vi "Initialize Modbus Slave Connection.vi"(8 "error in (no error)":errorcluster, 11 "Parameters":T1={"Interface Data"={"Name"="", "Unit ID"=0, "Refresh Rate"=0, "Write Rate"=0, "Write Mode"=enum."Value Change", "Interface Type"=enum."TCP Master", "TCP Settings"={"Address"="", "Port"=0, "Timeout"=0}, "Serial Settings"={"VISA resource name"="", "baud rate"=0, "parity (even)"=0, "flow control (none)"=0, "serial type"=enum."RTU", "Wire Mode"=-1}}, "Modbus Input Groups"=[], "Modbus Output Groups"=[], "error in (no error)"={"status"=FALSE, "code"=0, "source"=""}, "Modbus Input Engine Group Names"=[], "Modbus Output Engine Group Names"=[]} {"Interface Data"."Serial Settings"."Wire Mode" items=["Unknown"=-1, "RS485/Wire4"=0, "RS485/Wire2-EchoDTR"=1, "RS485/Wire2-CtrlDTR"=2, "RS485/Wire2-Auto"=3, "RS232/DTE"=128, "RS232/DCE"=129, "RS232/AUTO"=130]; "Interface Data"."Serial Settings"."parity (even)" items=["None", "Odd", "Even", "Mark", "Space"]; "Interface Data"."Serial Settings"."flow control (none)" items=["None", "XON/XOFF", "RTS/CTS", "XON/XOFF & RTS/CTS", "DTR/DSR", "XON/XOFF & DTR/DSR"]}) -> (0 "error out":errorcluster, 3 "Modbus Slave Out":refnum<class "Modbus Slave.lvclass">)   [LabVIEW 2021, in "Modbus Master Engine.lvlib"]
uses:
  Modbus Master Engine.lvlib
  Shared/Device Info.ctl
  Shared/Write Mode.ctl
  Shared/Controls/Interface Type.ctl
  Shared/Controls/Data Model/TCP Settings.ctl
  Shared/Controls/Data Model/Serial Settings.ctl
  Bulk Data Access.ctl
  System Explorer/SubVIs/Modbus Type.ctl
  Shared/Controls/Data Model/Channel.ctl
  <vilib>/NI VeriStand/Custom Device API/Custom Device Channel Type.ctl
  Shared/Controls/Data Model/Mapping.ctl
  Shared/Controls/Data Model/DataType.ctl
  <vilib>/NI VeriStand/Custom Device API/Custom Device Item Ref.ctl
  Modbus API.lvlibp/API/Slave/Modbus Slave.lvclass
  Modbus API.lvlibp/API/Wrapper/API Main.lvlib
  Shared/Modbus Master Shared.lvlib
  <vilib>/NI VeriStand/Custom Device API/Custom Device API.lvlib
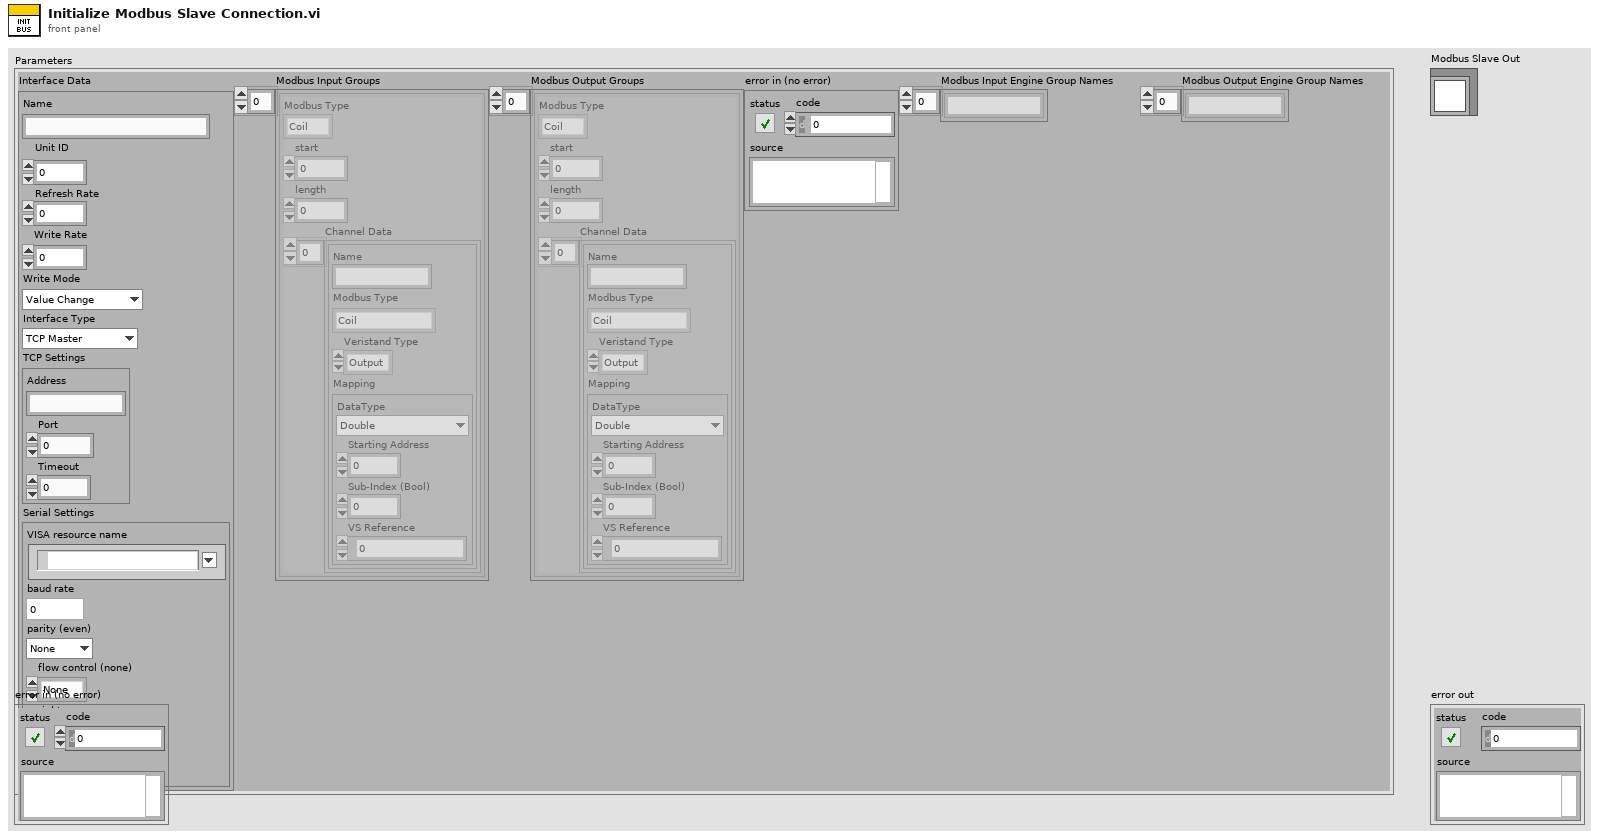
[diagram p1: front panel]
types:
  T1 = typedef "Modbus Master Shared.lvlib/Device Info.ctl" = cluster{"Interface Data":cluster{"Name":string, "Unit ID":u8, "Refresh Rate":i32, "Write Rate":i32, "Write Mode":T2, "Interface Type":T3, "TCP Settings":T4, "Serial Settings":T5}, "Modbus Input Groups":T6[], "Modbus Output Groups":T6[], "error in (no error)":errorcluster, "Modbus Input Engine Group Names":string[], "Modbus Output Engine Group Names":string[]}
  T2 = typedef "Modbus Master Shared.lvlib/Write Mode.ctl" = enum16{"Value Change", "Interval"}
  T3 = typedef "Modbus Master Shared.lvlib/Interface Type.ctl" = enum16{"TCP Master", "Serial Master", "TCP Slave", "Serial Slave"}
  T4 = typedef "Modbus Master Shared.lvlib/TCP Settings.ctl" = cluster{"Address":string, "Port":u16, "Timeout":i32}
  T5 = typedef "Modbus Master Shared.lvlib/Serial Settings.ctl" = cluster{"VISA resource name":refnum<visa-resource-name>, "baud rate":u32, "parity (even)":u16, "flow control (none)":u16, "serial type":enum16{"RTU", "ASCII"}, "Wire Mode":i16}
  T6 = typedef "Modbus Master Shared.lvlib/Bulk Data Access.ctl" = cluster{"Modbus Type":T7, "start":u16, "length":u16, "Channel Data":T8[]}
  T7 = typedef "Modbus Master Shared.lvlib/Modbus Type.ctl" = enum16{"Coil", "Discrete Input", "Holding Register", "Input Register"}
  T8 = typedef "Modbus Master Shared.lvlib/Channel.ctl" = cluster{"Name":string, "Modbus Type":T7, "Veristand Type":T9, "Mapping":T10}
  T9 = typedef "Custom Device API.lvlib/Custom Device Channel Type.ctl" = enum16{"Input", "Output"}
  T10 = typedef "Modbus Master Shared.lvlib/Mapping.ctl" = cluster{"DataType":T11, "Starting Address":u16, "Sub-Index (Bool)":u16, "VS Reference":T12}
  T11 = typedef "Modbus Master Shared.lvlib/DataType.ctl" = enum16{"Double", "Single", "I64", "I32", "I16", "I8", "U64", "U32", "U16", "U8", "Boolean"}
  T12 = typedef "Custom Device API.lvlib/Custom Device Item Ref.ctl" = u64
  T13 = cluster{"serial slave instances":refnum<class "Modbus Slave.lvclass">[], "VISA Resources":refnum<visa-resource-name>[]}
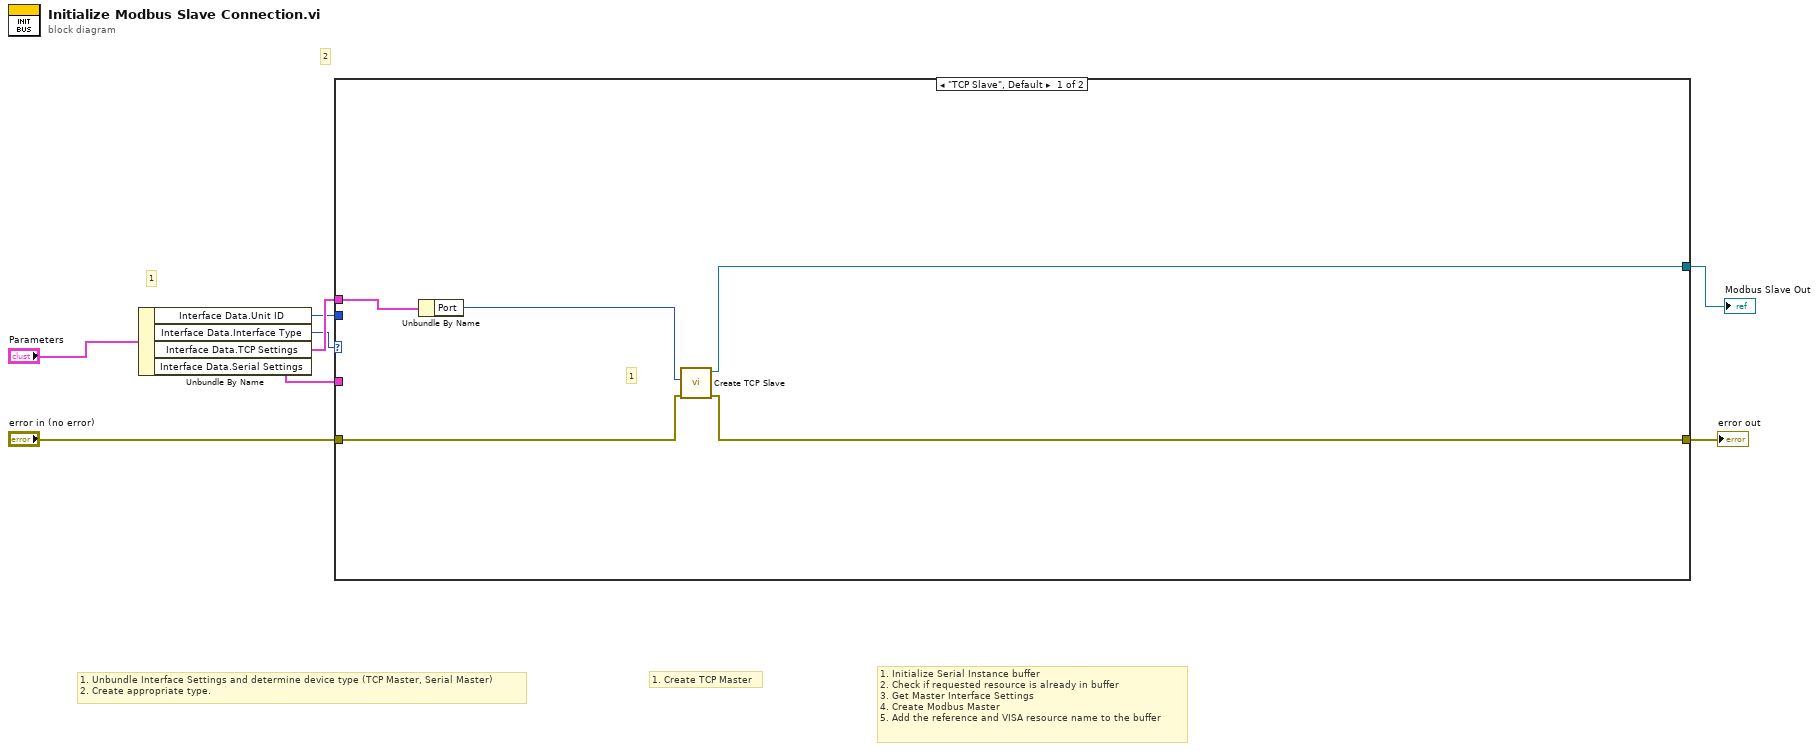
[diagram p0: block diagram]
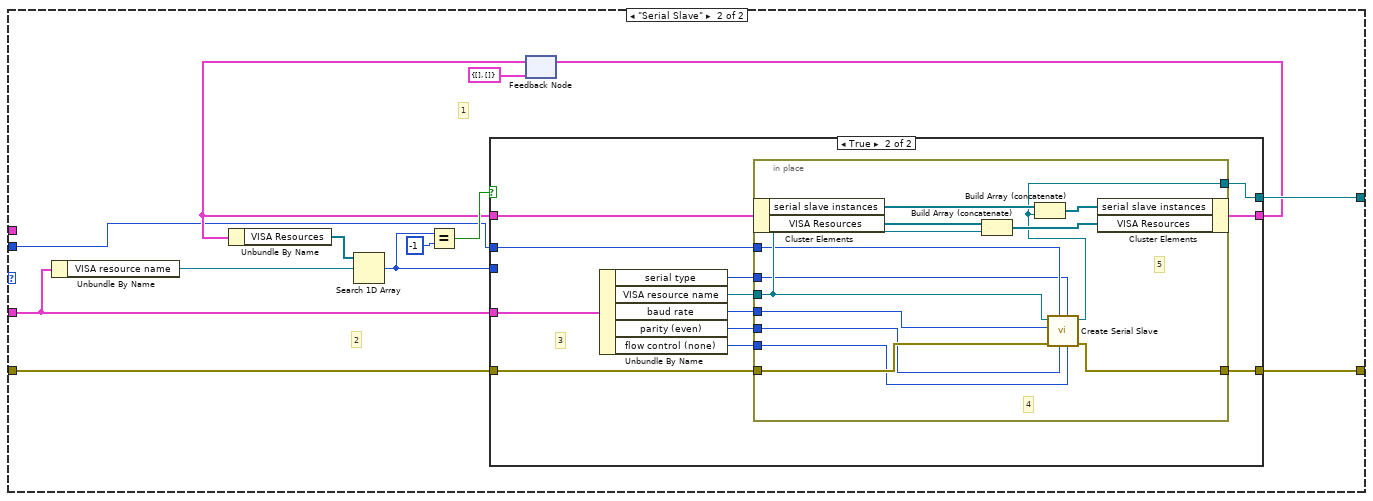
[diagram p2: hidden frame]
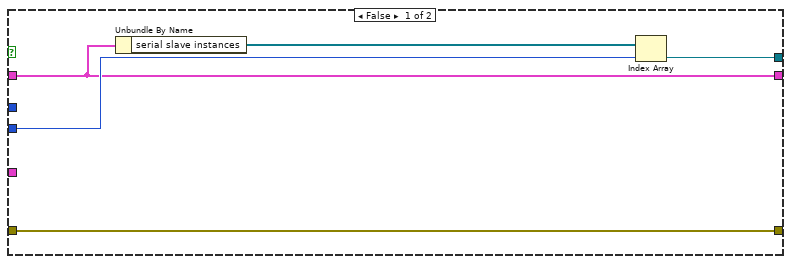
[diagram p3: hidden frame]
diagram:
  # "1. Initialize Serial Instance buffer\n2. Check if requested resource is already in buffer\n3. Get Master Interface Settings\n4. Create Modbus Master\n5. Add the reference and VISA resource name to the buffer"
  # "1. Create TCP Master"
  # "2"
  # "1"
  # "1. Unbundle Interface Settings and determine device type (TCP Master, Serial Master)\n2. Create appropriate type."
  n1 = Unbundle By Name("Parameters") -> ("Interface Data.Unit ID"=w1:u8, "Interface Data.Interface Type"=w6:T3, "Interface Data.TCP Settings"=w7:T4, "Interface Data.Serial Settings"=w8:T5)
  n2 = case shown="\"TCP Slave\", Default" w6 {
    tunnel: w7 -> [w13 _]
    tunnel: w8 -> [_ w15]
    tunnel: [w9 w24] -> w2
    tunnel: [w10 w26] -> w4
    tunnel: "error in (no error)" -> [w11 w25]
    tunnel: w1 -> [_ w14]
    frame "TCP Slave", Default {
      # "1"
      n3 = Unbundle By Name(w13) -> ("Port"=w12:u16)
      n4 = call "Create TCP Slave.vi"("error in"=w11, "port (502)"=w12) -> ("error out"=w10:errorcluster, "TCP slave instance"=w9:refnum<class "Modbus Slave.lvclass">)  [unwired: 8 in]
    }
    frame "Serial Slave" {
      # "2"
      # "1"
      n5 = Unbundle By Name(w15) -> ("VISA resource name"=w23:refnum<visa-resource-name>)
      n6 = feedback #1(T13 {"serial slave instances"=[], "VISA Resources"=[]}) -> (w18:T13)
      n7 = Unbundle By Name(w18) -> ("VISA Resources"=w17:refnum<visa-resource-name>[])
      n8 = Search 1D Array(1D array=w17, element=w23) -> (index of element=w20:i32)  [unwired: 1 in]
      n9 = Equal?(x=w20, y=-1) -> (x = y?=w21:bool)
      n10 = case shown="True" w21 {
        tunnel: [w30 w43] -> w26
        tunnel: w25 -> [w30 w42]
        tunnel: [w28 w41] -> w24
        tunnel: w20 -> [w31 _]
        tunnel: w18 -> [w27 w40]
        tunnel: [w27 w39] -> w16
        tunnel: w15 -> [_ w38]
        tunnel: w14 -> [_ w32]
        frame False {
          n11 = Unbundle By Name(w27) -> ("serial slave instances"=w29:refnum<class "Modbus Slave.lvclass">[])
          n12 = Index Array(array=w29, index=w31) -> (element=w28:refnum<class "Modbus Slave.lvclass">)
        }
        frame True {
          # "3"
          n13 = Unbundle By Name(w38) -> ("serial type"=w37:enum16{"RTU", "ASCII"}, "VISA resource name"=w36:refnum<visa-resource-name>, "baud rate"=w35:u32, "parity (even)"=w34:u16, "flow control (none)"=w33:u16)
          n14 = in-place {
            in-place-border: [w47] -> w43
            in-place-border: w42 -> [w56]
            in-place-border: [w44] -> w41
            in-place-border: w37 -> [w49]
            in-place-border: w36 -> [w51]
            in-place-border: w35 -> [w48]
            in-place-border: w34 -> [w46]
            in-place-border: w33 -> [w45]
            in-place-border: w32 -> [w50]
            # "5"
            # "4"
            n15 = in-place-cluster #2(w40) -> ("serial slave instances"=w53:refnum<class "Modbus Slave.lvclass">[], "VISA Resources"=w55:refnum<visa-resource-name>[])
            n16 = Build Array (concatenate)(w55, w51) -> (w54:refnum<visa-resource-name>[])
            n17 = call "Create Serial Slave.vi"("flow control"=w45, "serial type"=w49, "parity (even)"=w46, "unit ID"=w50, "error in"=w56, "baud rate (9600)"=w48, "VISA resource name"=w51) -> ("error out"=w47:errorcluster, "serial slave instance"=w44:refnum<class "Modbus Slave.lvclass">)  [unwired: 3 in]
            n18 = Build Array (concatenate)(w53, w44) -> (w52:refnum<class "Modbus Slave.lvclass">[])
            n19 = in-place-cluster #2("serial slave instances"=w52, "VISA Resources"=w54) -> (w39:T13)
          }
        }
      }
      n20 = feedback-in #1(w16) -> ()
    }
  }
  "error out" <- w4
  "Modbus Slave Out" <- w2
